vi "VI Reference To IWin32Window Reference.vi"(8 "error in (no error)":errorcluster, 10 "WindowWrapper DLL Directory":path, 11 "VI Reference":refnum<vi>) -> (0 "error out":errorcluster, 3 "System.Windows.Forms.IWin32Window":refnum<k24>)   [LabVIEW 2013, in "Win32 Util.lvlib"]
doc: "This VI obtains a IWin32Window Reference for the VI Front Panel that is specified by the VI Reference."
uses:
  Win32 Util.lvlib
  System.Windows.Forms
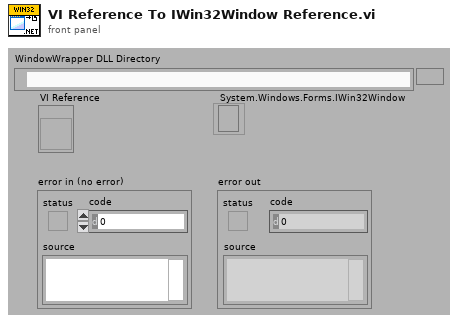
[diagram p1: front panel]
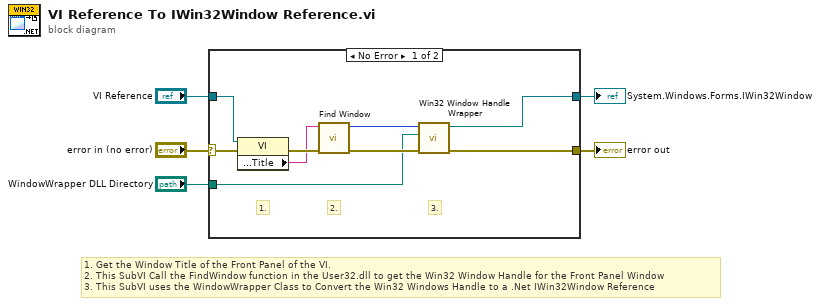
[diagram p0: block diagram]
diagram:
  # "1. Get the Window Title of the Front Panel of the VI.\n2. This SubVI Call the FindWindow function in the User32.dll to get the Win32 Window Handle for the Front Panel Window\n3. This SubVI uses the WindowWrapper Class to Convert the Win32 Windows Handle to a .Net IWin32Window Reference"
  n1 = case shown="No Error" "error in (no error)" {
    selector: "error in (no error)" -> [w7 w15]
    tunnel: [w14 _] -> w5
    tunnel: "VI Reference" -> [w9 _]
    tunnel: [w8 w15] -> w3
    tunnel: "WindowWrapper DLL Directory" -> [w6 _]
    frame No Error {
      # "3."
      # "2."
      # "1."
      n2 = property class="VI"(reference=w9, error in=w7) -> (error out=w11:errorcluster, "Front Panel.Title"=w10:string)  [unwired: 1 out]
      n3 = call "Find Window.vi"("error in (no error)"=w11, "Window Name"=w10) -> ("error out"=w13:errorcluster, "Win32 Window Handle"=w12:i32)  [unwired: 8 in]
      n4 = call "Win32 Window Handle Wrapper.vi"("error in (no error)"=w13, "WindowWrapper DLL Directory"=w6, "Win32 Window Handle"=w12) -> ("error out"=w8:errorcluster, "System.Windows.Forms.IWin32Window"=w14:refnum<k24>)  [unwired: 7 in]
    }
    frame Error {
    }
  }
  "System.Windows.Forms.IWin32Window" <- w5
  "error out" <- w3
